vi "Tray_SetTray_M.vi"(0 "TrayIn":refnum<vi>, 5 "GridSize":cluster{"x":u32, "y":u32}={"x"=6, "y"=16}, 7 "Index Number":i32=1, 9 "String":string, 11 "error in":errorcluster, 12 "Direction":u16=2, 13 "Color Box":u32(colorbox)=16448250) -> (15 "error out":errorcluster)   [LabVIEW 2019]
panel:
  out "TrayIn":cluster{"Color":u32[][], "Data":string[][]}={"Color"=[[16777215, 16777215, 16777215, 16777215, 16777215, 16777215], [16777215, 16777215, 16777215, 16777215, 16777215, 16777215], [16777215, 16777215, 16777215, 16777215, 16777215, 16777215], [16777215, 16777215, 16777215, 16777215, 16777215, 16777215], [16777215, 16777215, 16777215, 16777215, 16777215, 16777215], [16777215, 16777215, 16777215, 16777215, 16777215, 16777215], [16777215, 16777215, 16777215, 16777215, 16777215, 16777215], [16777215, 16777215, 16777215, 16777215, 16777215, 16777215], [16777215, 16777215, 16777215, 16777215, 16777215, 16777215], [16777215, 16777215, 16777215, 16777215, 16777215, 16777215], [16777215, 16777215, 16777215, 16777215, 16777215, 16777215], [16777215, 16777215, 16777215, 16777215, 16777215, 16777215], [16777215, 16777215, 16777215, 16777215, 16777215, 16777215], [16777215, 16777215, 16777215, 16777215, 16777215, 16777215], [16777215, 16777215, 16777215, 16777215, 16777215, 16777215], [16777215, 16777215, 16777215, 16777215, 16777215, 16777215]], "Data"=[["91", "92", "93", "94", "95", "96"], ["85", "86", "87", "88", "89", "90"], ["79", "80", "81", "82", "83", "84"], ["73", "74", "75", "76", "77", "78"], ["67", "68", "69", "70", "71", "72"], ["61", "62", "63", "64", "65", "66"], ["55", "56", "57", "58", "59", "60"], ["49", "50", "51", "52", "53", "54"], ["43", "44", "45", "46", "47", "48"], ["37", "38", "39", "40", "41", "42"], ["31", "32", "33", "34", "35", "36"], ["25", "26", "27", "28", "29", "30"], ["19", "20", "21", "22", "23", "24"], ["13", "14", "15", "16", "17", "18"], ["7", "8", "9", "10", "11", "12"], ["1", "2", "3", "4", "5", "6"]]}
  # "Start Index is 1"
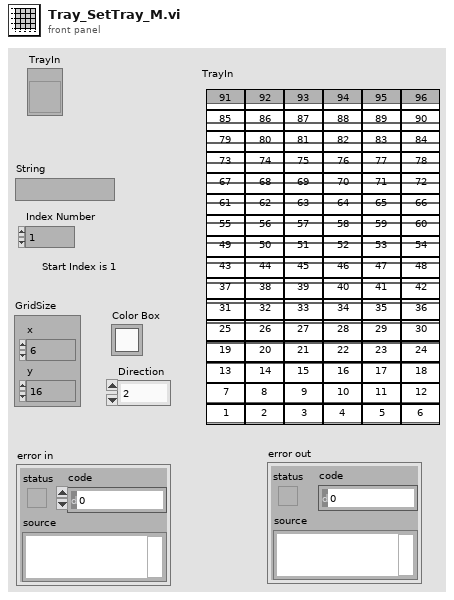
[diagram p1: front panel]
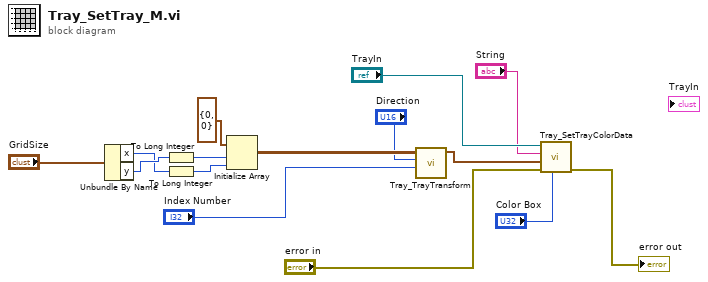
[diagram p0: block diagram]
diagram:
  n1 = Unbundle By Name("GridSize") -> ("x"=w11:u32, "y"=w12:u32)
  n2 = To Long Integer(number=w12) -> (32bit integer=w14:i32)
  n3 = To Long Integer(number=w11) -> (32bit integer=w15:i32)
  n4 = Initialize Array(cluster{"X":i32, "Y":i32} {"X"=0, "Y"=0} ("Cluster"), w14, w15) -> (w9:cluster{"X":i32, "Y":i32}[][])
  n5 = call "Tray_TrayTransform.vi"("StartNumber"="Index Number", "Direction"="Direction", "TrayIn"=w9) -> ("ArrayIndex"=w6:cluster{"X":i32, "Y":i32})  [unwired: 8 in]
  n6 = call "Tray_SetTrayColorData.vi"("Color"="Color Box", "error in (no error)"="error in", "Index"=w6, "Data"="String", "TrayRef"="TrayIn") -> ("error out"=→"error out":errorcluster)  [unwired: 6 in]
